vi "1-7.vi"() -> ()   [LabVIEW 2022 SP3]
panel:
  in  "数值输入控件":dbl
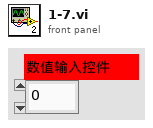
[diagram p1: front panel]
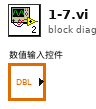
[diagram p0: block diagram]
diagram:
